vi "UserInterface_Main.vi"(3 "error in (no error)":errorcluster) -> (10 "error out":errorcluster)   [LabVIEW 2020]
uses:
  Controller/#typedef_ControllerQueue_States.ctl
  Cmd_enum.ctl
  #typedef_UserInterface_Data.ctl
  #typedef_Parameters_cluster.ctl
  BaudRate_enum.ctl
  Controller/#typedef_Controller_Data.ctl
  <vilib>/Instr/_visa.llb/VISA Configure Serial Port (Instr).vi
panel:
  in  "Read data":bool
  in  "Baud Rate":enum32{"9600", "115200"}(ring)
  in  "Serial Port":refnum<visa-resource-name>="N/A"
  out "Logs":string
  out "Chart":dbl(graph)
  in  "Stop":bool
  in  "Disconnect":bool
  in  "Connect":bool
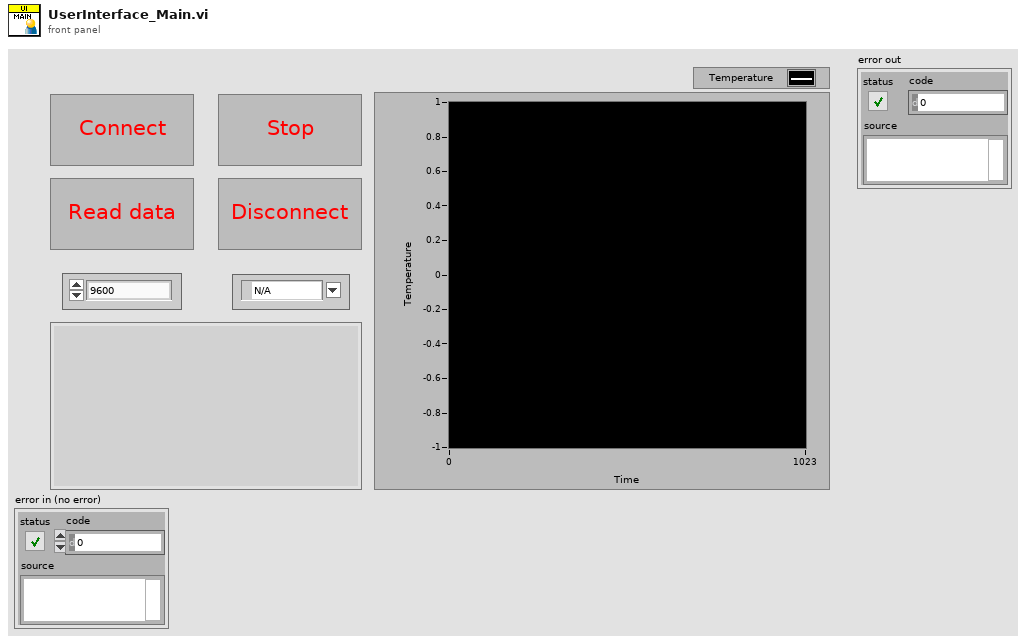
[diagram p1: front panel]
types:
  T1 = typedef "#typedef_ControllerQueue_States.ctl" = enum16{"Obtain", "GetRef", "Enqueue", "EnqueueAtOpp", "GetStatus", "Flush", "Release"}
  T2 = typedef "BaudRate_enum.ctl" = enum16{"115200", "9600"}
  T3 = typedef "#typedef_UserInterface_Data.ctl" = cluster{"Cmd":T4, "Param":T5, "Temperature":dbl, "Logs":string}
  T4 = typedef "Cmd_enum.ctl" = enum16{"Init", "PrintChart", "Connect", "Disconnect", "ReadData", "Exit"}
  T5 = typedef "#typedef_Parameters_cluster.ctl" = cluster{"Stop":bool, "Connect":bool, "Disconnect":bool, "Port COM":refnum<visa-resource-name>, "Baud rate":T2}
  T6 = typedef "#typedef_Controller_Data.ctl" = cluster{"Cmd":enum16{"Idle", "PrintChart", "SendToDB", "Exit"}, "Temperature":dbl, "Logs":string}
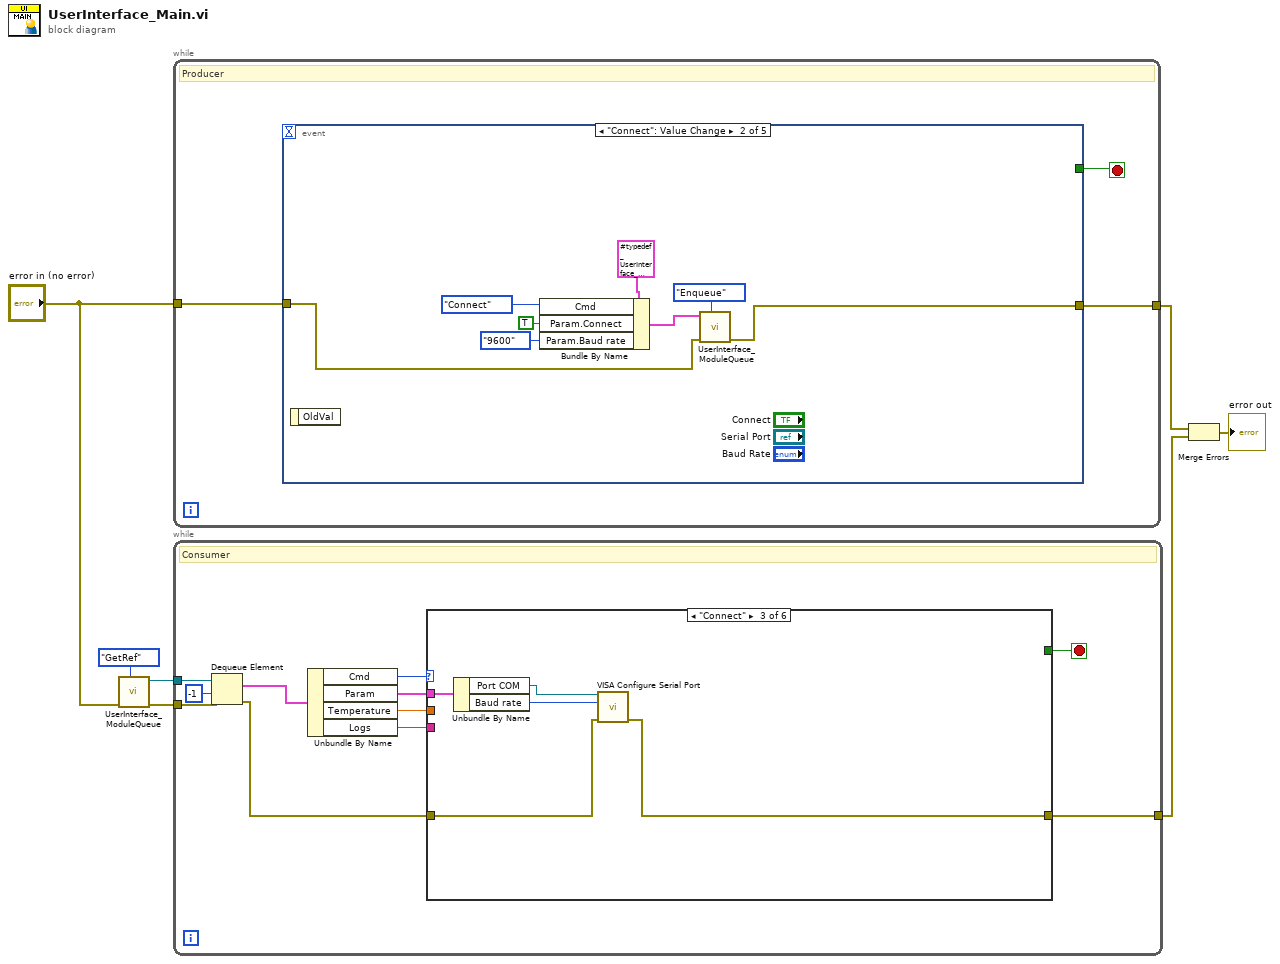
[diagram p0: block diagram]
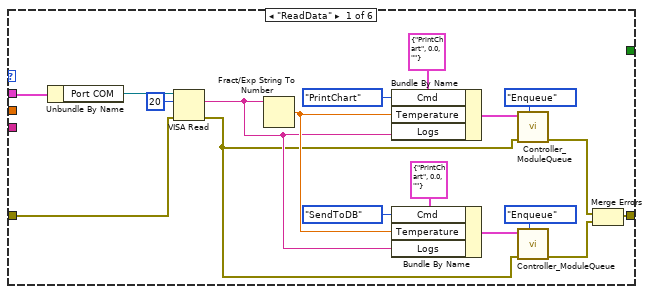
[diagram p2: hidden frame]
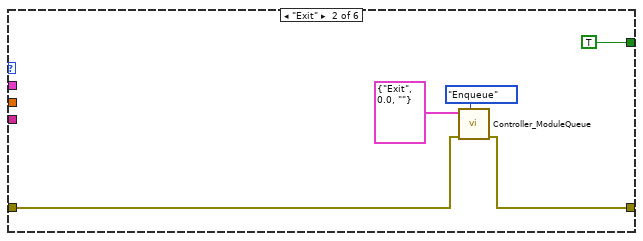
[diagram p3: hidden frame]
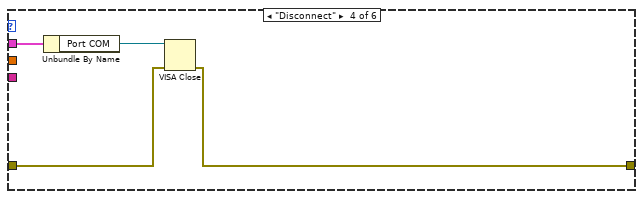
[diagram p4: hidden frame]
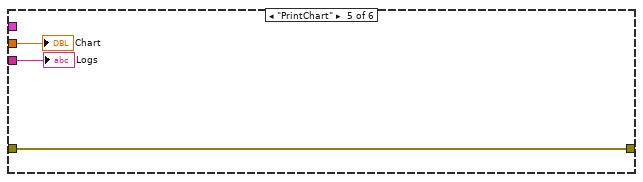
[diagram p5: hidden frame]
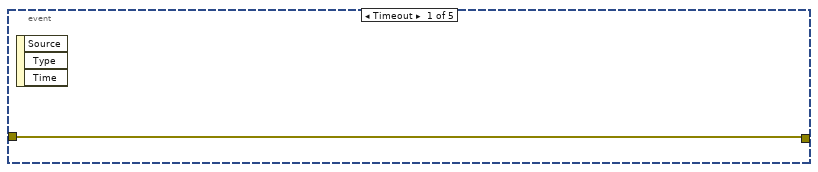
[diagram p7: hidden frame]
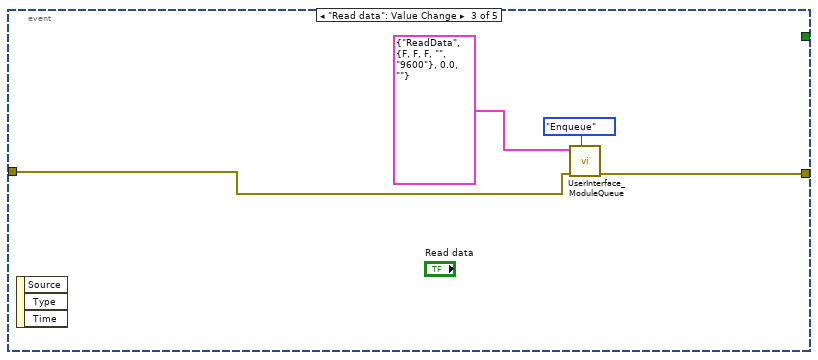
[diagram p8: hidden frame]
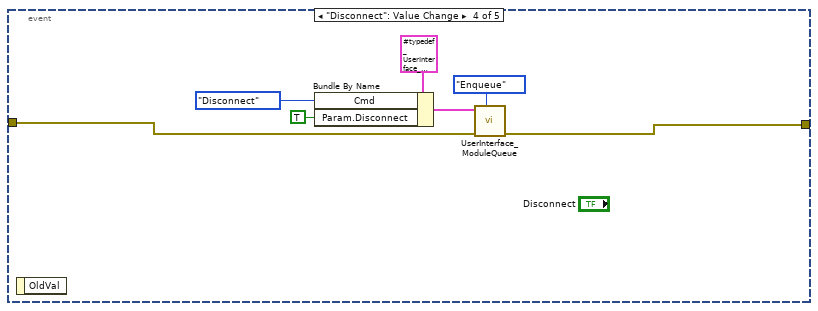
[diagram p9: hidden frame]
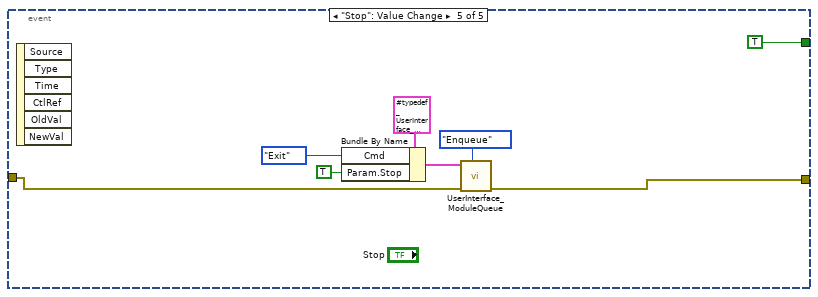
[diagram p10: hidden frame]
diagram:
  n1 = call "UserInterface_ModuleQueue.vi"(7:#typedef_ControllerQueue_States."GetRef", "error in (no error)"="error in (no error)") -> ("error out"=w6:errorcluster, "queue out"=w1:refnum<queue>)  [unwired: 7 in, 1 out]
  n2 = while {
    tunnel: "error in (no error)" -> [w9]
    tunnel: [w8] -> w4
    stop <- w10 stop-if-true
    # "Producer"
    n3 = event shown="[1] \"Connect\": Value Change" {
      selector: _ -> [_ _ _ _ _]
      dyn-events: _ -> [_ _ _ _ _]
      timeout: _ -> [_ _ _ _ _]
      tunnel: [_ _ _ _ TRUE] -> w10
      tunnel: w9 -> [w11 w16 w22 w27 w34]
      tunnel: [w11 w15 w21 w26 w33] -> w8
      event Timeout {
        n4 = event-data() -> ()  [unwired: 1 in, 3 out]
      }
      event "Connect": Value Change {
        n5 = event-data() -> ()  [unwired: 1 in, 1 out]
        n6 = Bundle By Name(cluster=T3 {"Cmd"=enum."Init", "Param"={"Stop"=FALSE, "Connect"=FALSE, "Disconnect"=FALSE, "Port COM"="", "Baud rate"=enum."115200"}, "Temperature"=0.0, "Logs"=""} ("ToConsumentData"), "Cmd"=Cmd_enum."Connect", "Param.Connect"=TRUE, "Param.Baud rate"=BaudRate_enum."9600") -> (w13:T3)
        n7 = call "UserInterface_ModuleQueue.vi"(7:#typedef_ControllerQueue_States."Enqueue", "error in (no error)"=w16, "DataIn"=w13) -> ("error out"=w15:errorcluster)  [unwired: 6 in, 2 out]
      }
      event "Read data": Value Change {
        n8 = event-data() -> ()  [unwired: 1 in, 3 out]
        n9 = call "UserInterface_ModuleQueue.vi"(7:#typedef_ControllerQueue_States."Enqueue", "error in (no error)"=w22, "DataIn"=T3 {"Cmd"=enum."ReadData", "Param"={"Stop"=FALSE, "Connect"=FALSE, "Disconnect"=FALSE, "Port COM"="", "Baud rate"=enum."9600"}, "Temperature"=0.0, "Logs"=""}) -> ("error out"=w21:errorcluster)  [unwired: 6 in, 2 out]
      }
      event "Disconnect": Value Change {
        n10 = event-data() -> ()  [unwired: 1 in, 1 out]
        n11 = Bundle By Name(cluster=T3 {"Cmd"=enum."Init", "Param"={"Stop"=FALSE, "Connect"=FALSE, "Disconnect"=FALSE, "Port COM"="", "Baud rate"=enum."115200"}, "Temperature"=0.0, "Logs"=""} ("DataIn"), "Cmd"=Cmd_enum."Disconnect", "Param.Disconnect"=TRUE ("Param.Stop")) -> (w24:T3)
        n12 = call "UserInterface_ModuleQueue.vi"(7:#typedef_ControllerQueue_States."Enqueue", "error in (no error)"=w27, "DataIn"=w24) -> ("error out"=w26:errorcluster)  [unwired: 6 in, 2 out]
      }
      event "Stop": Value Change {
        n13 = event-data() -> ()  [unwired: 1 in, 6 out]
        n14 = Bundle By Name(cluster=T3 {"Cmd"=enum."Init", "Param"={"Stop"=FALSE, "Connect"=FALSE, "Disconnect"=FALSE, "Port COM"="", "Baud rate"=enum."115200"}, "Temperature"=0.0, "Logs"=""} ("DataIn"), "Cmd"=Cmd_enum."Exit", "Param.Stop"=TRUE) -> (w31:T3)
        n15 = call "UserInterface_ModuleQueue.vi"(7:#typedef_ControllerQueue_States."Enqueue", "error in (no error)"=w34, "DataIn"=w31) -> ("error out"=w33:errorcluster)  [unwired: 6 in, 2 out]
      }
    }
  }
  n16 = while {
    tunnel: w6 -> [w46]
    tunnel: [w44] -> w3
    tunnel: w1 -> [w41]
    stop <- w47 stop-if-true
    # "Consumer"
    n17 = Dequeue Element(queue=w41, timeout in ms (-1)=-1, error in (no error)=w46) -> (element=w42:T3, error out=w45:errorcluster)  [unwired: 2 out]
    n18 = Unbundle By Name(w42) -> ("Cmd"=w49:T4, "Param"=w48:T5, "Temperature"=w39:dbl, "Logs"=w40:string)
    n19 = case shown="\"Connect\"" w49 {
      tunnel: w48 -> [w67 _ w75 w81 _ _]
      tunnel: [_ TRUE _ _ _ _] -> w47
      tunnel: w45 -> [w64 w70 w77 w80 w84 w85]
      tunnel: [w52 w69 w76 w79 w84 w85] -> w44
      tunnel: w40 -> [_ _ _ _ w83 _]
      tunnel: w39 -> [_ _ _ _ w82 _]
      frame "ReadData" {
        n20 = Unbundle By Name(w67) -> ("Port COM"=w66:refnum<visa-resource-name>)
        n21 = VISA Read(VISA resource name=w66, byte count=u32 20, error in (no error)=w64) -> (read buffer=w56:string, error out=w55:errorcluster)  [unwired: 2 out]
        n22 = Fract/Exp String To Number(string=w56) -> (number=w57:dbl)  [unwired: 3 in, 1 out]
        n23 = Bundle By Name(cluster=T6 {"Cmd"=enum."PrintChart", "Temperature"=0.0, "Logs"=""} ("Data in"), "Cmd"=enum16{"Idle", "PrintChart", "SendToDB", "Exit"}."PrintChart", "Temperature"=w57, "Logs"=w56) -> (w61:T6)
        n24 = Bundle By Name(cluster=T6 {"Cmd"=enum."PrintChart", "Temperature"=0.0, "Logs"=""} ("Data in"), "Cmd"=enum16{"Idle", "PrintChart", "SendToDB", "Exit"}."SendToDB", "Temperature"=w57, "Logs"=w56) -> (w58:T6)
        n25 = call "Controller_ModuleQueue.vi"(7:#typedef_ControllerQueue_States."Enqueue", "error in (no error)"=w55, "Data in"=w61) -> ("error out"=w54:errorcluster)  [unwired: 6 in, 2 out]
        n26 = call "Controller_ModuleQueue.vi"(7:#typedef_ControllerQueue_States."Enqueue", "error in (no error)"=w55, "Data in"=w58) -> ("error out"=w53:errorcluster)  [unwired: 6 in, 2 out]
        n27 = Merge Errors(w54, w53) -> (w52:errorcluster)
      }
      frame "Exit" {
        n28 = call "Controller_ModuleQueue.vi"(7:#typedef_ControllerQueue_States."Enqueue", "error in (no error)"=w70, "Data in"=T6 {"Cmd"=enum."Exit", "Temperature"=0.0, "Logs"=""}) -> ("error out"=w69:errorcluster)  [unwired: 6 in, 2 out]
      }
      frame "Connect" {
        n29 = Unbundle By Name(w75) -> ("Port COM"=w74:refnum<visa-resource-name>, "Baud rate"=w73:T2)
        n30 = call-poly "VISA Configure Serial Port"("VISA resource name"=w74, "baud rate (9600)"=w73, "error in (no error)"=w77) -> ("error out"=w76:errorcluster)  [unwired: 11 in, 1 out]
      }
      frame "Disconnect" {
        n31 = Unbundle By Name(w81) -> ("Port COM"=w78:refnum<visa-resource-name>)
        n32 = VISA Close(VISA resource name=w78, error in (no error)=w80) -> (error out=w79:errorcluster)
      }
      frame "PrintChart" {
        "Chart" <- w82
        "Logs" <- w83
      }
      frame "Init" {
      }
    }
  }
  n33 = Merge Errors(w4, w3) -> (→"error out":errorcluster)
